vi "PointLineDistance.vi"(1 "LinePoint2":T1, 2 "LinePoint1":T1, 3 "TestPoint":T1) -> (0 "Distance":dbl)   [LabVIEW 2017]
uses:
  PathPlanning/TypeDefs/Point2D.ctl
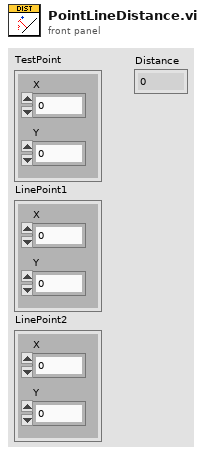
[diagram p1: front panel]
types:
  T1 = typedef "Point2D.ctl" = cluster{"X":dbl, "Y":dbl}
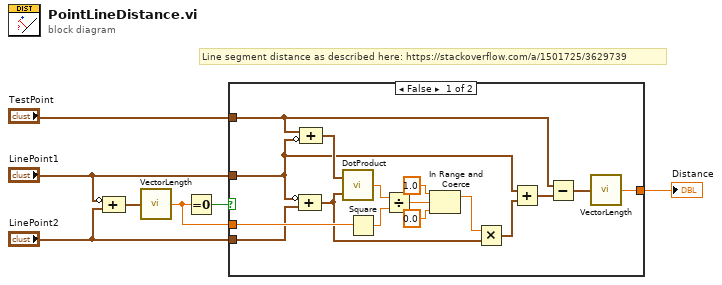
[diagram p0: block diagram]
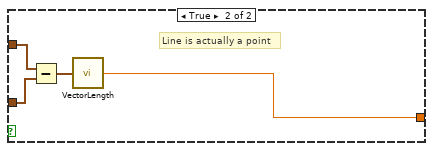
[diagram p2: hidden frame]
diagram:
  # "Line segment distance as described here: https://stackoverflow.com/a/1501725/3629739"
  n1 = Compound Arithmetic op=ADD(invert "LinePoint1", "LinePoint2") -> (w7:T1)
  n2 = call "VectorLength.vi"("VectorIn"=w7) -> ("VectorLength"=w3:dbl)
  n3 = Equal To 0?(x=w3) -> (x = 0?=w6:bool)
  n4 = case shown="False" w6 {
    tunnel: "LinePoint1" -> [w12 w26]
    tunnel: "LinePoint2" -> [w17 _]
    tunnel: "TestPoint" -> [w10 w27]
    tunnel: [w8 w24] -> w4
    tunnel: w3 -> [w23 _]
    frame False {
      n5 = Compound Arithmetic op=ADD(invert w12, w17) -> (w14:T1)
      n6 = Compound Arithmetic op=ADD(w10, invert w12) -> (w16:T1)
      n7 = call "DotProduct.vi"("Y"=w14, "X"=w16) -> ("X*Y"=w20:dbl)
      n8 = Square(x=w23) -> (x^2=w19:dbl)
      n9 = Divide(x=w20, y=w19) -> (x/y=w18:dbl)
      n10 = In Range and Coerce(upper limit=1.0, x=w18, lower limit=0.0) -> (coerced(x)=w15:dbl)  [unwired: 1 out]
      n11 = Multiply(x=w15, y=w14) -> (x*y=w13:T1)
      n12 = Add(x=w12, y=w13) -> (x+y=w11:T1)
      n13 = Subtract(x=w10, y=w11) -> (x-y=w9:T1)
      n14 = call "VectorLength.vi"("VectorIn"=w9) -> ("VectorLength"=w8:dbl)
    }
    frame True {
      # "Line is actually a point"
      n15 = Subtract(x=w27, y=w26) -> (x-y=w25:T1)
      n16 = call "VectorLength.vi"("VectorIn"=w25) -> ("VectorLength"=w24:dbl)
    }
  }
  "Distance" <- w4
